vi "LV front desct.vi"(7 "Boolean":bool, 10 "Controls[]":refnum<vi>[](array[refnum]), 11 "All Objects[]":refnum<vi>[](array[refnum])) -> (3 "front":string)   [LabVIEW 2012]
panel:
  in  "vi path":path
  out "controls":T1(array[cluster])
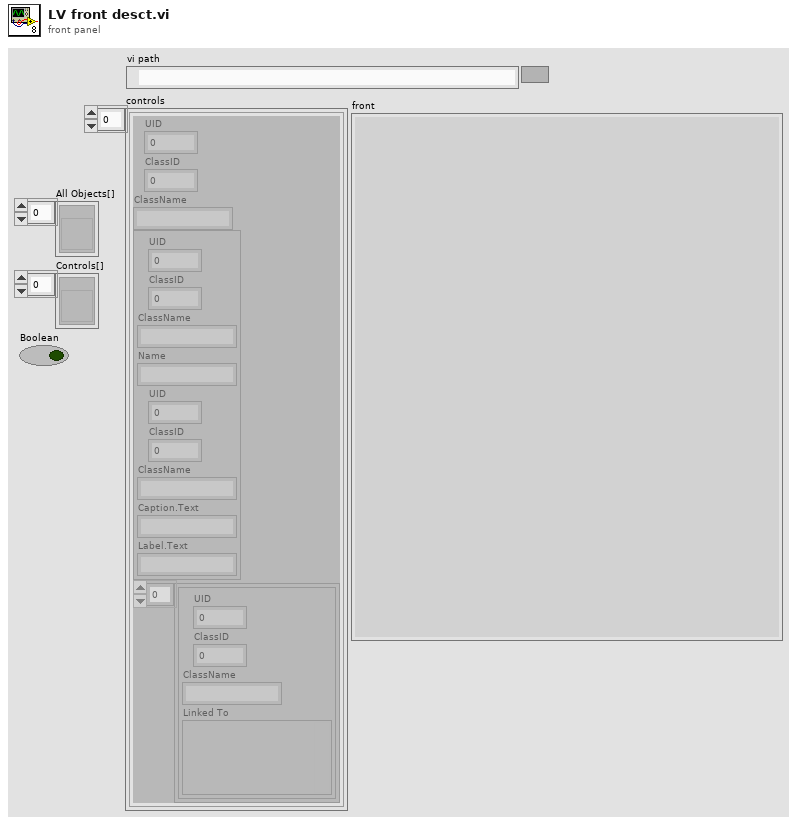
[diagram p1: front panel]
types:
  T1 = cluster{"UID":i32, "ClassID":u32, "ClassName":string, cluster{"UID":i32, "ClassID":u32, "ClassName":string, "Name":string, "UID":i32, "ClassID":u32, "ClassName":string, "Caption.Text":string, "Label.Text":string}, cluster{"UID":i32, "ClassID":u32, "ClassName":string, "Linked To":variant}[]}[]
  T2 = cluster{"UID":i32, "ClassID":u32, "ClassName":string, "Linked To":variant}
  T3 = cluster{"UID":i32, "ClassID":u32, "ClassName":string, "Name":string, "UID":i32, "ClassID":u32, "ClassName":string, "Caption.Text":string, "Label.Text":string}
  T4 = cluster{"UID":i32, "ClassName":string, "ClassName":string, cluster{"UID":i32, "ClassID":u32, "ClassName":string, "Name":string, "UID":i32, "ClassID":u32, "ClassName":string, "Caption.Text":string, "Label.Text":string}, cluster{"UID":i32, "ClassID":u32, "ClassName":string, "Linked To":variant}[]}
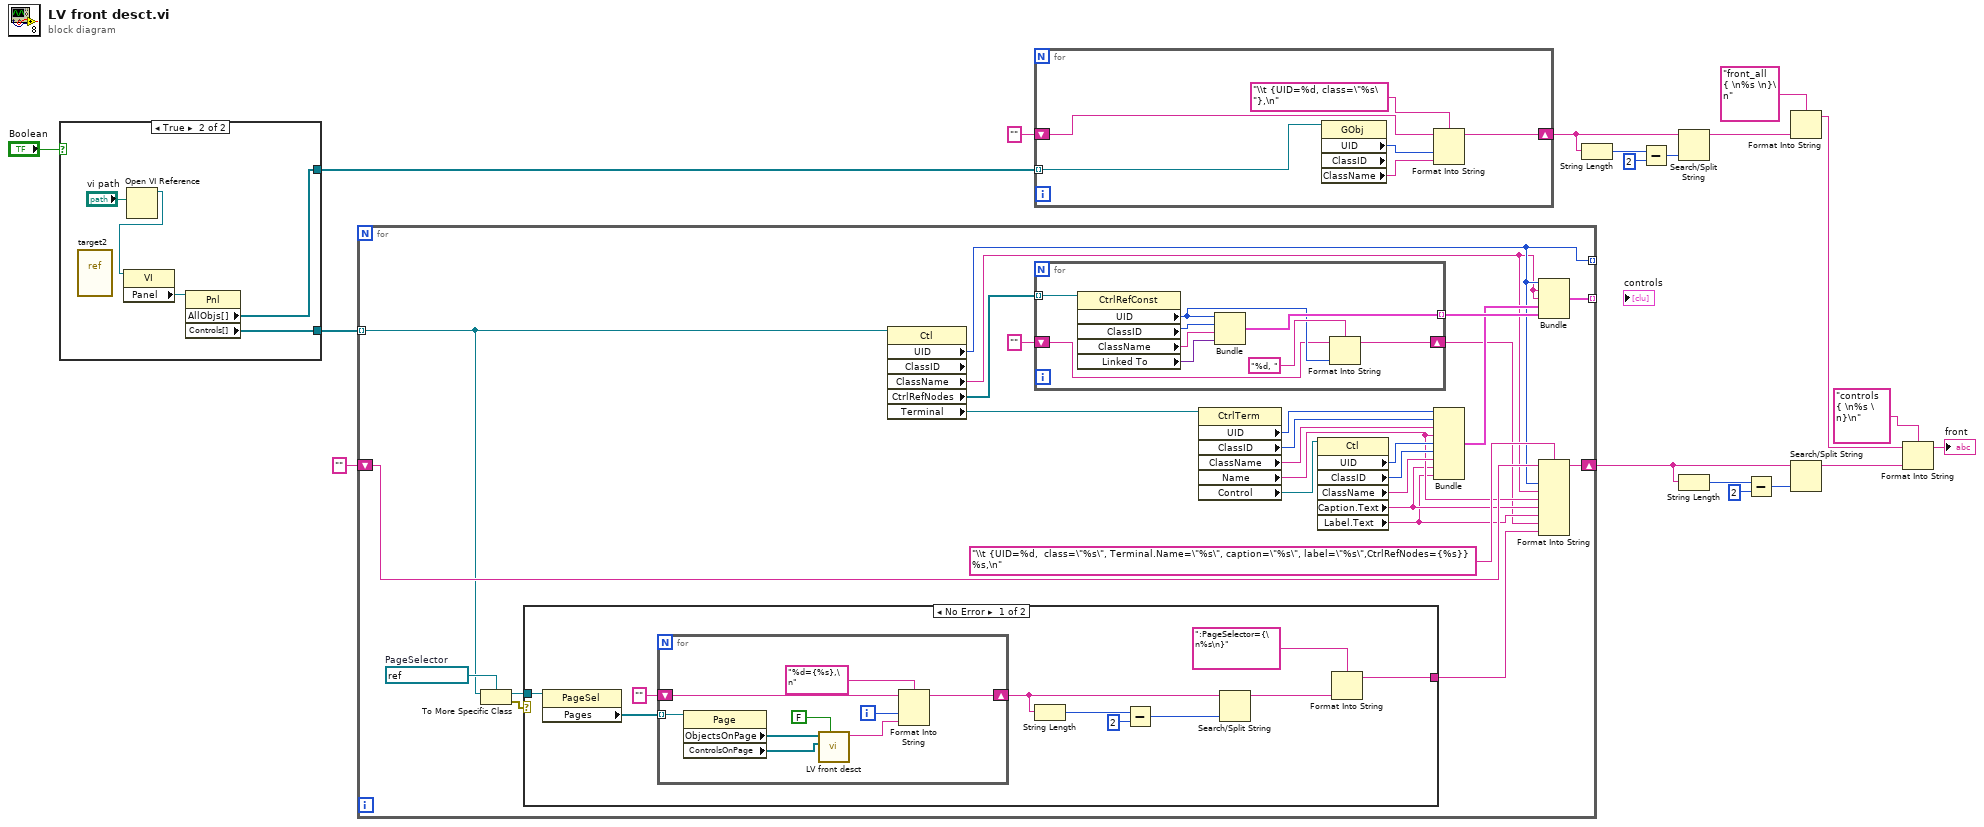
[diagram p0: block diagram]
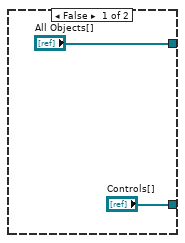
[diagram p2: hidden frame]
diagram:
  n1 = case shown="True" "Boolean" {
    tunnel: ["Controls[]" w26] -> w19
    tunnel: ["All Objects[]" w24] -> w18
    frame False {
    }
    frame True {
      n2 = vi-ref "target2.vi"() -> ()  [unwired: 1 out]
      n3 = Open VI Reference(vi path="vi path") -> (vi reference=w22:refnum<vi>)  [unwired: 5 in, 1 out]
      n4 = property class="VI"(reference=w22) -> ("Panel"=w25:refnum<vi>)  [unwired: 1 in, 2 out]
      n5 = property class="Pnl"(reference=w25) -> ("AllObjs[]"=w24:refnum<vi>[], "Controls[]"=w26:refnum<vi>[])  [unwired: 1 in, 2 out]
    }
  }
  n6 = for {
    tunnel: w19 -> [w32] mode=indexing
    tunnel: [w53] -> _ mode=indexing
    tunnel: [w39] -> _ mode=indexing
    shift-right: [w38] -> w6
    shift-left: "" -> [w41]
    w33 = refnum<vi> refnum  # PageSelector
    n7 = To More Specific Class(target class=w33, reference=w32) -> (specific class reference=w30:refnum<vi>, error out=w31:errorcluster)  [unwired: 1 in]
    n8 = case shown="No Error" w31 {
      tunnel: w30 -> [w63 _]
      tunnel: [w59 _] -> w29
      frame No Error {
        n9 = property class="PageSel"(reference=w63) -> ("Pages"=w62:refnum<vi>[])  [unwired: 1 in, 2 out]
        n10 = for {
          tunnel: w62 -> [w72] mode=indexing
          shift-right: [w68] -> w55
          shift-left: "" -> [w67]
          i -> [w64]
          n11 = property class="Page"(reference=w72) -> ("ObjectsOnPage"=w71:refnum<vi>[], "ControlsOnPage"=w70:refnum<vi>[])  [unwired: 1 in, 2 out]
          n12 = call "LV front desct.vi"("Boolean"=FALSE, "Controls[]"=w70, "All Objects[]"=w71) -> ("front"=w65:string)  [unwired: 8 in]
          n13 = Format Into String(format string="%d={%s},\n", initial string=w67, w64, w65) -> (resulting string=w68:string)  [unwired: 1 in, 1 out]
        }
        n14 = String Length(string=w55) -> (length=w56:i32)
        n15 = Subtract(x=w56, y=2) -> (x-y=w58:i32)
        n16 = Search/Split String(string=w55, offset (0)=w58) -> (substring before match=w54:string)  [unwired: 1 in, 2 out]
        n17 = Format Into String(format string=":PageSelector={\n%s\n}", w54) -> (resulting string=w59:string)  [unwired: 2 in, 1 out]
      }
      frame Error {
      }
    }
    n18 = property class="Ctl" props=["UID", "ClassID", "ClassName", "CtrlRefNodes", "Terminal"](reference=w32) -> ("UID"=w39:i32, "ClassName"=w27:string, "CtrlRefNodes"=w51:refnum<vi>[], "Terminal"=w50:refnum<vi>)  [unwired: 1 in, 3 out]
    n19 = for {
      tunnel: w51 -> [w81] mode=indexing
      tunnel: [w78] -> w52 mode=indexing
      shift-right: [w74] -> w28
      shift-left: "" -> [w73]
      n20 = property class="CtrlRefConst"(reference=w81) -> ("UID"=w75:i32, "ClassID"=w80:u32, "ClassName"=w79:string, "Linked To"=w77:variant)  [unwired: 1 in, 2 out]
      n21 = Bundle("UID"=w75, "ClassID"=w80, "ClassName"=w79, "Linked To"=w77) -> (w78:T2)  [unwired: 1 in]
      n22 = Format Into String(format string="%d, ", initial string=w73, w75) -> (resulting string=w74:string)  [unwired: 1 in, 1 out]
    }
    n23 = property class="CtrlTerm"(reference=w50) -> ("UID"=w48:i32, "ClassID"=w47:u32, "ClassName"=w46:string, "Name"=w37:string, "Control"=w49:refnum<vi>)  [unwired: 1 in, 2 out]
    n24 = property class="Ctl"(reference=w49) -> ("UID"=w45:i32, "ClassID"=w44:u32, "ClassName"=w43:string, "Caption.Text"=w36:string, "Label.Text"=w35:string)  [unwired: 1 in, 2 out]
    n25 = Bundle("UID"=w48, "ClassID"=w47, "ClassName"=w46, "Name"=w37, "UID"=w45, "ClassID"=w44, "ClassName"=w43, "Caption.Text"=w36, "Label.Text"=w35) -> (w42:T3)  [unwired: 1 in]
    n26 = Bundle("UID"=w39, "ClassName"=w27, "ClassName"=w27, w42, w52) -> (w53:T4)  [unwired: 1 in]
    n27 = Format Into String(format string="\\t {UID=%d,  class=\"%s\", Terminal.Name=\"%s\", caption=\"%s\", label=\"%s\",CtrlRefNodes={%s}} %s,\n", initial string=w41, w39, w27, w37, w36, w35, w28, w29) -> (resulting string=w38:string)  [unwired: 1 in, 1 out]
  }
  n28 = for {
    tunnel: w18 -> [w87] mode=indexing
    shift-right: [w83] -> w12
    shift-left: "" -> [w84]
    n29 = property class="GObj" props=["UID", "ClassID", "ClassName"](reference=w87) -> ("UID"=w86:i32, "ClassName"=w82:string)  [unwired: 1 in, 3 out]
    n30 = Format Into String(format string="\\t {UID=%d, class=\"%s\"},\n", initial string=w84, w86, w82) -> (resulting string=w83:string)  [unwired: 1 in, 1 out]
  }
  n31 = String Length(string=w12) -> (length=w15:i32)
  n32 = Subtract(x=w15, y=2) -> (x-y=w13:i32)
  n33 = Search/Split String(string=w12, offset (0)=w13) -> (substring before match=w11:string)  [unwired: 1 in, 2 out]
  n34 = String Length(string=w6) -> (length=w7:i32)
  n35 = Subtract(x=w7, y=2) -> (x-y=w9:i32)
  n36 = Format Into String(format string="front_all { \n%s \n}\n", w11) -> (resulting string=w3:string)  [unwired: 2 in, 1 out]
  n37 = Search/Split String(string=w6, offset (0)=w9) -> (substring before match=w4:string)  [unwired: 1 in, 2 out]
  n38 = Format Into String(format string="controls { \n%s \n}\n", initial string=w3, w4) -> (resulting string=→"front":string)  [unwired: 1 in, 1 out]
